vi "Shifter.vi"(6 "SolenoidDevRef":T1, 9 "SolenoidDevRef 2":T1, 10 "ButtonShiftUp":bool, 11 "ButtonShiftDown":bool) -> ()   [LabVIEW 2015]
uses:
  <vilib>/Rock Robotics/WPI/Solenoid/WPI_SolenoidChannel.ctl
  <vilib>/Rock Robotics/WPI/Solenoid/WPI_SolenoidDevRef.ctl
panel:
  out "RightShift":bool=TRUE
  out "SolenoidDevRef 4":T1={"DevStatus"={"status"=FALSE, "code"=0, "source"=""}, "Pneumatics Control Module"=0, "Forward Solenoid Channel"=enum."Invalid", "Reverse Solenoid Channel"=enum."Invalid"}
  out "LeftShift":bool=TRUE
  out "SolenoidDevRef 3":T1={"DevStatus"={"status"=FALSE, "code"=0, "source"=""}, "Pneumatics Control Module"=0, "Forward Solenoid Channel"=enum."Invalid", "Reverse Solenoid Channel"=enum."Invalid"}
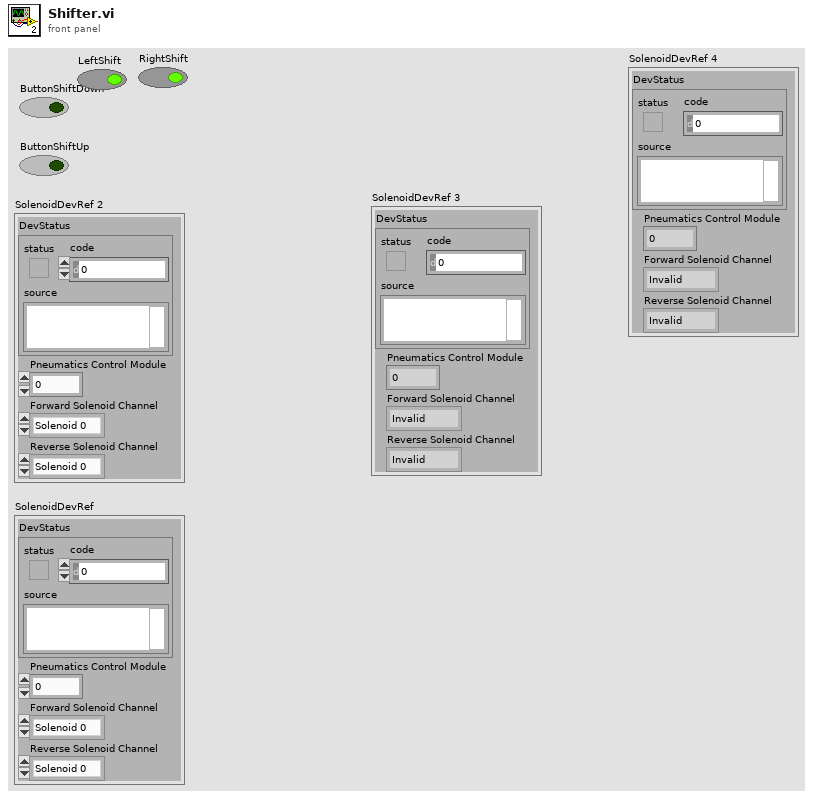
[diagram p1: front panel]
types:
  T1 = typedef "WPI_SolenoidDevRef.ctl" = cluster{"DevStatus":errorcluster, "Pneumatics Control Module":u8, "Forward Solenoid Channel":T2, "Reverse Solenoid Channel":T2}
  T2 = typedef "WPI_SolenoidChannel.ctl" = enum8{"Solenoid 0", "Solenoid 1", "Solenoid 2", "Solenoid 3", "Solenoid 4", "Solenoid 5", "Solenoid 6", "Solenoid 7", "Invalid"}
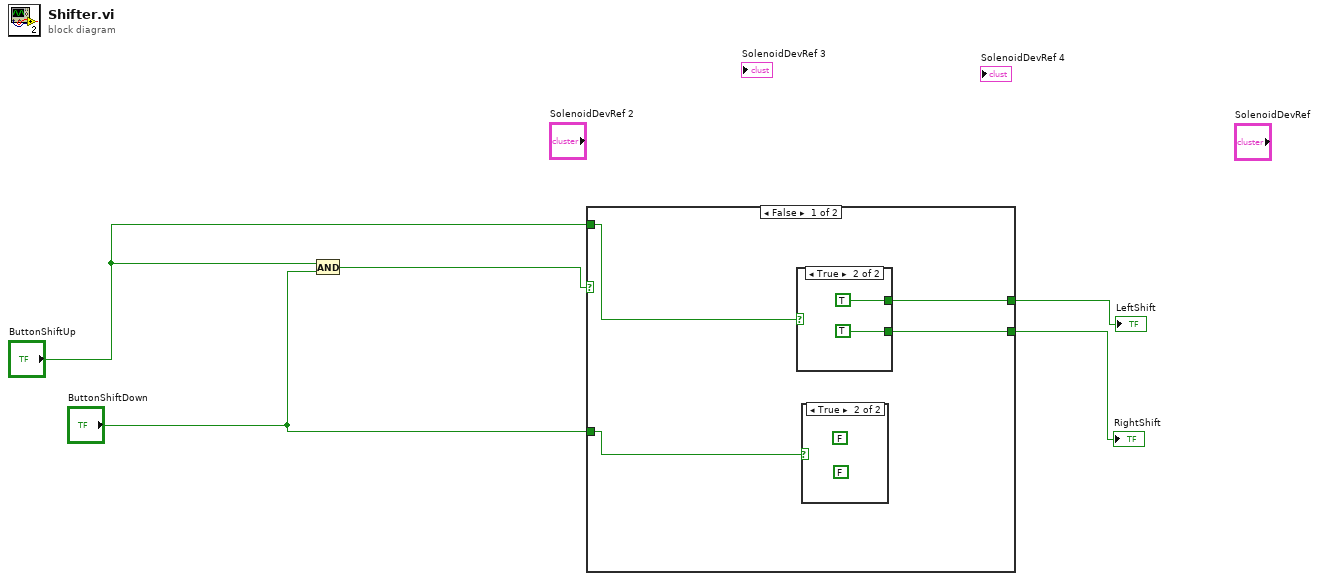
[diagram p0: block diagram]
diagram:
  n1 = And(x="ButtonShiftUp", y="ButtonShiftDown") -> (x .and. y?=w3:bool)
  n2 = case shown="False" w3 {
    tunnel: "ButtonShiftUp" -> [w9 _]
    tunnel: "ButtonShiftDown" -> [w8 _]
    tunnel: [w7 _] -> w2
    tunnel: [w6 _] -> w1
    frame False {
      n3 = case shown="True" w9 {
        tunnel: [_ TRUE] -> w7
        tunnel: [_ TRUE] -> w6
        frame False {
        }
        frame True {
        }
      }
      n4 = case shown="True" w8 {
        frame False {
        }
        frame True {
          (unwired) FALSE
          (unwired) FALSE
        }
      }
    }
    frame True {
    }
  }
  "LeftShift" <- w2
  "RightShift" <- w1
